vi "Init Data.vi"(10 "Data":T1) -> (3 "Msg out":refnum<class "Msg.lvclass">)   [LabVIEW 2020, in "UdpPayload.lvlib" / "Msg.lvclass"]
uses:
  Msg.lvclass
  Data.ctl
  UdpPayload.lvlib
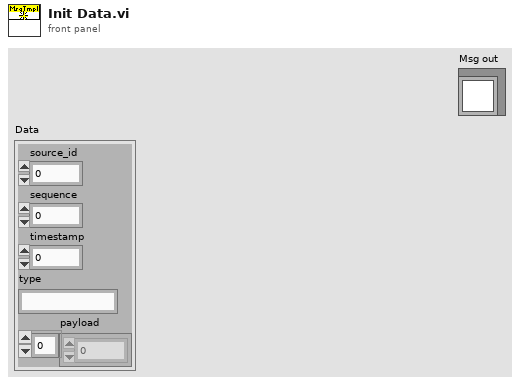
[diagram p1: front panel]
types:
  T1 = typedef "UdpPayload.lvlib/Data.ctl" = cluster{"source_id":u32, "sequence":u32, "timestamp":i64, "type":string, "payload":u8[]}
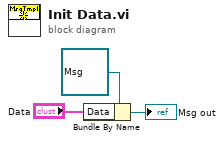
[diagram p0: block diagram]
diagram:
  n1 = Bundle By Name(cluster=refnum<class "Msg.lvclass"> refnum ("Msg out"), "Data"="Data") -> (→"Msg out":refnum<class "Msg.lvclass">)
